vi "Update Distance To Wall Using Encoders.vi"(11 "Period (ms)":dbl) -> (3 "Wall Distance":dbl(graph)=592.5)   [LabVIEW 2017]
uses:
  Globals/Pose.vi
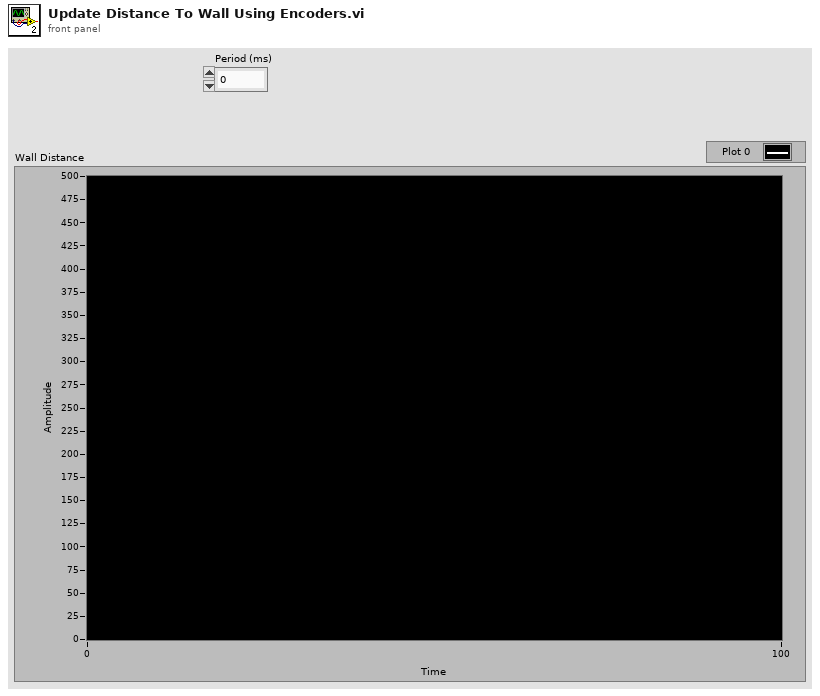
[diagram p1: front panel]
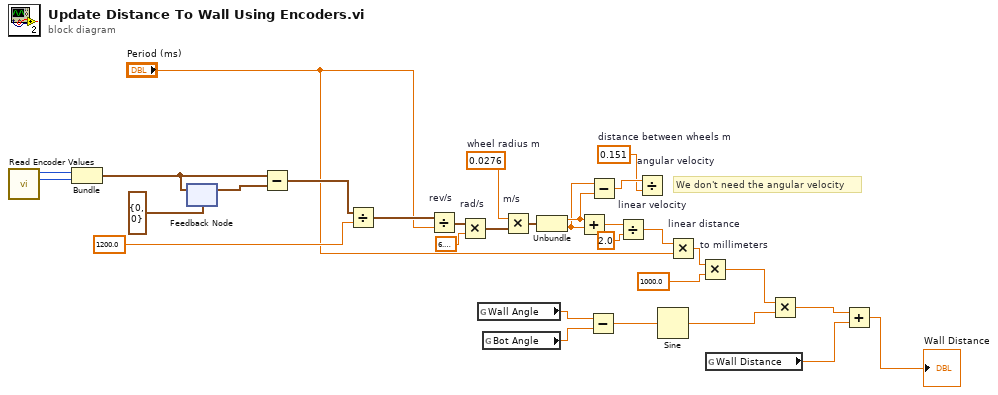
[diagram p0: block diagram]
diagram:
  w21 = 0.151  # distance between wheels m
  w29 = 0.0276  # wheel radius m
  # "We don't need the angular velocity"
  n1 = call "Read Encoder Values.vi"() -> ("Right Value"=w13:i32, "Left  Value"=w14:i32)  [unwired: 10 in]
  n2 = Bundle("Left  Value"=w14, "Right Value"=w13) -> (w18:cluster{"Left  Value":i32, "Right Value":i32})  [unwired: 1 in]
  n3 = feedback #1(cluster{"Left  Value":i32, "Right Value":i32} {"Left  Value"=0, "Right Value"=0}) -> (w19:cluster{"Left  Value":i32, "Right Value":i32})
  n4 = feedback-in #1(w18) -> ()
  n5 = Subtract(x=w18, y=w19) -> (x-y=w15:cluster{"Left  Value":i32, "Right Value":i32})
  n6 = Divide(x=w15, y=1200.0 ("Left  Value")) -> (x/y=w16:cluster{"Left  Value":dbl, "Right Value":dbl})
  n7 = Divide "rev/s"(x=w16, y="Period (ms)") -> (x/y=w31:cluster{"Left  Value":dbl, "Right Value":dbl})
  n8 = Multiply "rad/s"(x=w31, y=6.283185307179586) -> (x*y=w28:cluster{"Left  Value":dbl, "Right Value":dbl})
  n9 = global read "Pose.vi" "Wall Angle"() -> (w4:dbl)
  n10 = global read "Pose.vi" "Bot Angle"() -> (w3:dbl)
  n11 = Multiply "m/s"(x=w29, y=w28) -> (x*y=w25:cluster{"Left  Value":dbl, "Right Value":dbl})
  n12 = Unbundle(w25) -> ("Left  Value"=w24:dbl, "Right Value"=w23:dbl)
  n13 = Add(x=w24, y=w23) -> (x+y=w26:dbl)
  n14 = Subtract(x=w4, y=w3) -> (x-y=w11:dbl)
  n15 = Subtract(x=w23, y=w24) -> (x-y=w22:dbl)
  n16 = Divide "linear velocity"(x=w26, y=2.0) -> (x/y=w8:dbl)
  n17 = Divide "angular velocity"(x=w22, y=w21) -> ()  [unwired: 1 out]
  n18 = Sine(x=w11) -> (sin(x)=w12:dbl)
  n19 = Multiply "linear distance"(x=w8, y="Period (ms)") -> (x*y=w6:dbl)
  n20 = Multiply "to millimeters"(x=w6, y=1000.0) -> (x*y=w7:dbl)
  n21 = global read "Pose.vi" "Wall Distance"() -> (w9:dbl)
  n22 = Multiply(x=w7, y=w12) -> (x*y=w10:dbl)
  n23 = Add(x=w10, y=w9) -> (x+y=→"Wall Distance":dbl)
